vi "Hall_sensor_measurement.vi"() -> ()   [LabVIEW 2019]
panel:
  out "Waveform Chart":T1(graph)
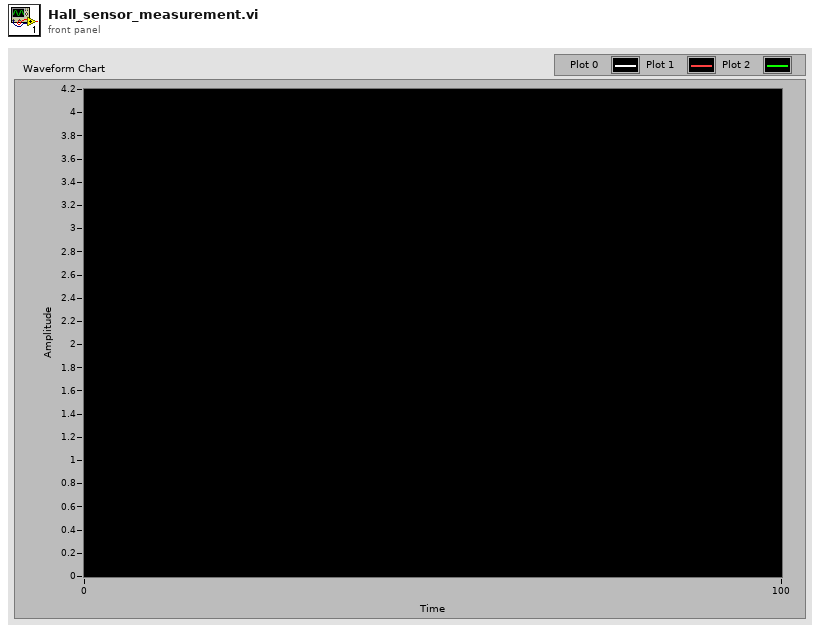
[diagram p1: front panel]
types:
  T1 = cluster{"[0]":dbl, "[1]":dbl, "[2]":dbl, "[3]":dbl, "[4]":dbl, "[5]":dbl, "[6]":dbl, "[7]":dbl, "[8]":dbl}
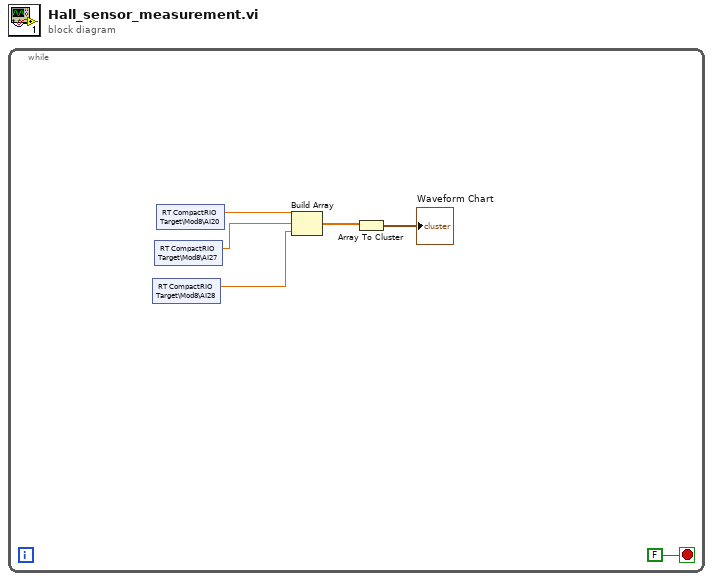
[diagram p0: block diagram]
diagram:
  n1 = while {
    stop <- FALSE stop-if-true
    n2 = shared-variable "RT CompactRIO Target\\Mod8\\AI28"() -> (w3:dbl)  [unwired: 1 in, 1 out]
    n3 = shared-variable "RT CompactRIO Target\\Mod8\\AI27"() -> (w4:dbl)  [unwired: 1 in, 1 out]
    n4 = shared-variable "RT CompactRIO Target\\Mod8\\AI20"() -> (w5:dbl)  [unwired: 1 in, 1 out]
    n5 = Build Array(w5, w4, w3) -> (w2:dbl[])
    n6 = Array To Cluster(array=w2) -> (cluster=→"Waveform Chart":T1)
  }
